vi "NextPtWrite2File 4.vi"(7 "Save the Graph":bool, 9 "Graph to be Saved":cluster{"Time":dbl[], "Peak-bkg Value":dbl[]}(graph), 10 "ProjectName":string="QFinger", 11 "Folder path input":path=path "C:/Labview34970A stuff/Data") -> (2 "Header":string, 3 "new file path that was created":path)   [LabVIEW 2016]
doc: "This takes a graph as input and writes it to a file. It grabs the column labels from the graph display.\nThe file naming is automated with DataFileCreator.vi\nDataFileCreator.vi is given an input Folder path and ProjectName this VI creates the next data file in the format \n2017-09-17ProjectName#001\nIt only checks the latest file in the folder to decide if \na sequence with today's date already exists.\nIf the file sequence has not been started, it creates one begining with #001\nIf it happens that it tries to create a file that already exists, a dialog pops up\nasking for a new name.\nAdd any comments you want saved in the file.\nPush the \"Save the Graph\" if you want the save to happen. This eliminates the need for the query in the main program."
uses:
  <vilib>/Utility/file.llb/Write To Spreadsheet File (DBL).vi
panel:
  in  "X,Y point to be added to file":dbl[](array[numeric])
  # "This takes a graph as input and writes it to a file. It grabs the column labels from the graph display.\nThe file naming is automated with DataFileCreator.vi\nDataFileCreator.vi is given an input Folder path and ProjectName this VI creates the next data file in the format \n2017-09-17ProjectName#001\nIt only checks the latest file in the folder to decide if \na sequence with today's date already exists.\nIf the file sequence has not been started, it creates one begining with #001\nIf it happens that it tries to create a file that already exists, a dialog pops up\nasking for a new name.\nAdd any comments you want saved in the file.\nPush the \"Save the Graph\" if you want the save to happen. This eliminates the need for the query in the main program."
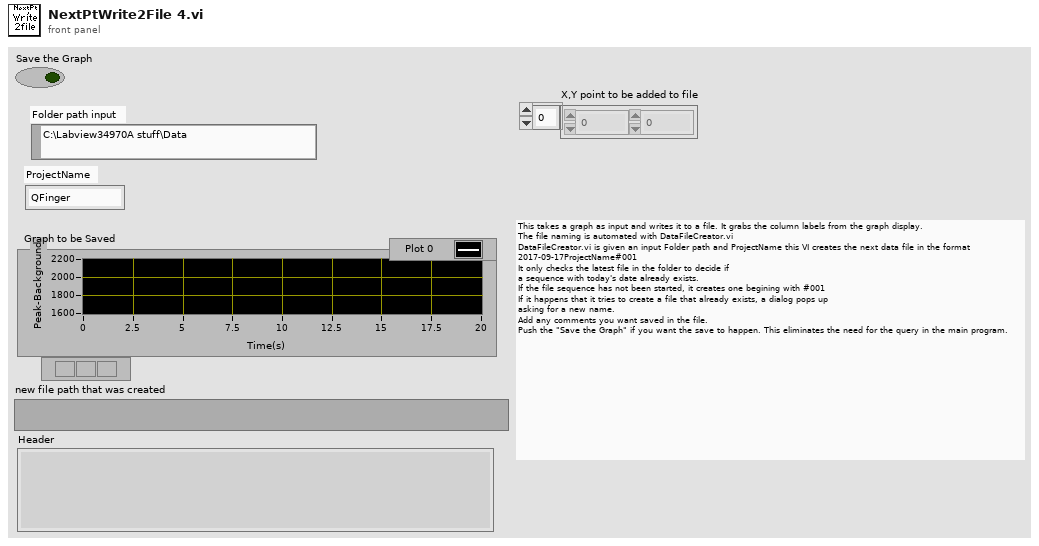
[diagram p1: front panel]
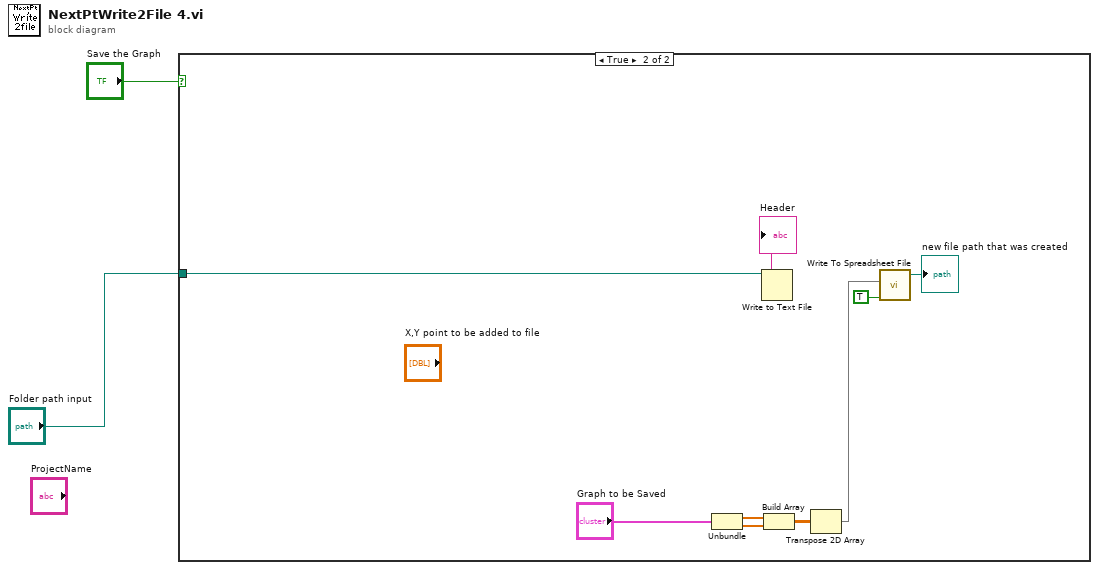
[diagram p0: block diagram]
diagram:
  n1 = case shown="True" "Save the Graph" {
    tunnel: "Folder path input" -> [_ w4]
    frame False {
    }
    frame True {
      n2 = Unbundle("Graph to be Saved") -> ("Time"=w6:dbl[], "Peak-bkg Value"=w5:dbl[])
      n3 = Write to Text File(file (use dialog)=w4, text="Header") -> ()  [unwired: 2 in, 3 out]
      n4 = Build Array(w6, w5) -> (w13:dbl[][])
      n5 = Transpose 2D Array(2D array=w13) -> (transposed array=w11:dbl[][])
      n6 = call-poly <vilib>:"Write To Spreadsheet File.vi"("append to file? (new file:F)"=TRUE, "2D data"=w11) -> ("new file path (Not A Path if cancelled)"=→"new file path that was created":path, "file path (dialog if empty)"=w8:path)  [unwired: 5 in]
    }
  }
